vi "Test Event Response.vi"   [LabVIEW 2015]
doc: "Drop this template to test the event response. If no event is fired within the timeout then the test fails.\n\nAdd handling cases for the event you expect."
uses:
  <vilib>/addons/_JKI Toolkits/VI Tester/TestCase.llb/TestCase.lvclass
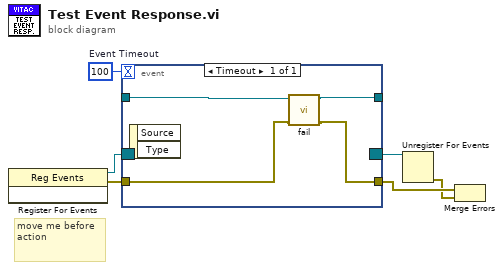
[diagram p0: block diagram]
diagram:
  w6 = 100  # Event Timeout
  # "move me before\naction"
  n1 = register-events() -> (reference out=w1:refnum<event-registration>, error out=w5:errorcluster)  [unwired: 3 in]
  n2 = event shown="[0] Timeout" {
    selector: w1 -> [_]
    dyn-events: [_] -> w4
    timeout: w6 -> [_]
    tunnel: _ -> [w10]
    tunnel: [w9] -> _
    tunnel: [w7] -> w3
    tunnel: w5 -> [w8]
    event Timeout {
      n3 = event-data() -> ()  [unwired: 1 in, 2 out]
      n4 = call-dynamic "fail.vi"("error in (no error)"=w8, "TestCase in"=w10) -> ("error out"=w7:errorcluster, "TestCase out"=w9:refnum<class "TestCase.lvclass">)  [unwired: 8 in]
    }
  }
  n5 = Unregister For Events(event registration refnum=w4) -> (error out=w2:errorcluster)  [unwired: 1 in]
  n6 = Merge Errors(w3, w2) -> ()  [unwired: 1 out]
